vi "SetUp.vi"(8 "error in (no error)":errorcluster, 11 "Prueba01 in":refnum<class "Prueba01.lvclass">) -> (0 "error out":errorcluster, 3 "Prueba01 out":refnum<class "Prueba01.lvclass">)   [LabVIEW 2019, in "Prueba01.lvclass"]
uses:
  Prueba01.lvclass
  Prueba01.lvclass/Prueba01.ctl
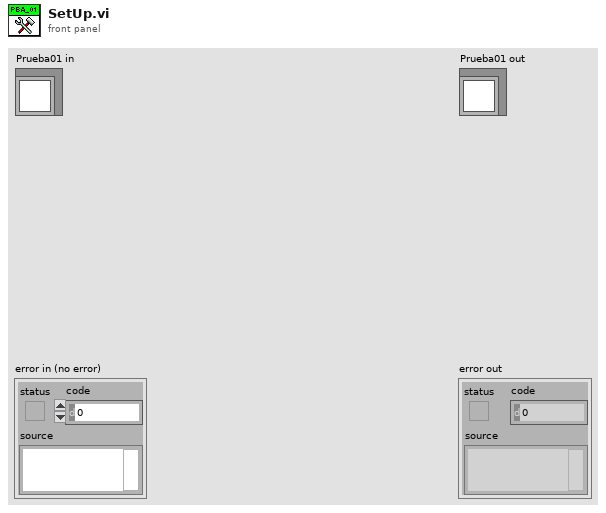
[diagram p1: front panel]
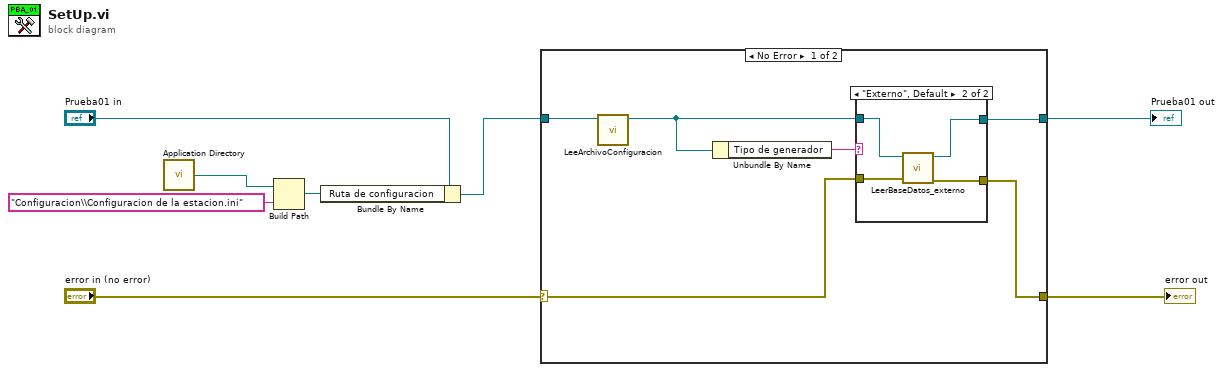
[diagram p0: block diagram]
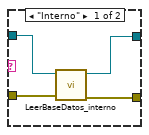
[diagram p2: hidden frame]
diagram:
  n1 = call <vilib>:"Application Directory.vi"() -> ("Application Directory"=w4:path)
  n2 = Build Path(base path=w4, name or relative path="Configuracion\\Configuracion de la estacion.ini") -> (appended path=w3:path)
  n3 = Bundle By Name(cluster="Prueba01 in", "Ruta de configuracion"=w3) -> (w1:refnum<class "Prueba01.lvclass">)
  n4 = case shown="No Error" "error in (no error)" {
    selector: "error in (no error)" -> [w14 w23]
    tunnel: w1 -> [w10 w24]
    tunnel: [w13 w24] -> w7
    tunnel: [w12 w23] -> w6
    frame No Error {
      n5 = call "LeeArchivoConfiguracion.vi"("Prueba01 in"=w10) -> ("Prueba01 out"=w9:refnum<class "Prueba01.lvclass">)  [unwired: 9 in, 1 out]
      n6 = Unbundle By Name(w9) -> ("Tipo de generador"=w11:string)
      n7 = case shown="\"Externo\", Default" w11 {
        tunnel: w14 -> [w18 w22]
        tunnel: [w17 w21] -> w13
        tunnel: [w16 w20] -> w12
        tunnel: w9 -> [w15 w19]
        frame "Interno" {
          n8 = call "LeerBaseDatos_interno.vi"("error in (no error)"=w18, "Prueba01 in"=w15) -> ("error out"=w16:errorcluster, "Prueba01 out"=w17:refnum<class "Prueba01.lvclass">)  [unwired: 8 in]
        }
        frame "Externo", Default {
          n9 = call "LeerBaseDatos_externo.vi"("error in (no error)"=w22, "Prueba01 in"=w19) -> ("error out"=w20:errorcluster, "Prueba01 out"=w21:refnum<class "Prueba01.lvclass">)  [unwired: 8 in]
        }
      }
    }
    frame Error {
    }
  }
  "error out" <- w6
  "Prueba01 out" <- w7
